vi "Drive Command Handler Temp.vi"(6 "Operator POVs":i16[](array[numeric]), 7 "Driver POVs":i16[](array[numeric]), 8 "Operator Axes":dbl[](array[numeric]), 9 "Operator Buttons":bool[](array[boolean]), 10 "Driver Buttons":bool[](array[boolean]), 11 "Driver Axes":dbl[](array[numeric])) -> ()   [LabVIEW 2019]
uses:
  Implementation/Drive Base Operations.ctl
  4946ced4-976c-43e8-b0b1-bcd015106e49.vi
  41fdccfd-133c-48c3-bd45-6bb0d7214a34.vi
  963458c1-dddb-4085-8820-b897a4c2a4ef.vi
  a950058a-1ddc-42d1-ab8e-bd80fb7a5a61.vi
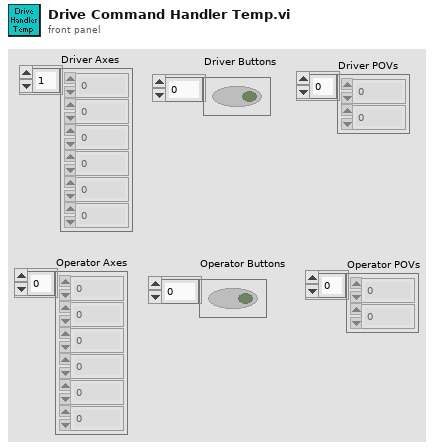
[diagram p1: front panel]
types:
  T1 = typedef "Drive Base Operations.ctl" = enum16{"Reserve", "Read Current", "Immediate", "Immediate Limelight", "Immediate Duration", "Limelight", "Manual Adjustment", "Play Path"}
  T2 = cluster{"f":T1, "Cluster":cluster{"Numeric":dbl, "Numeric 2":dbl}}
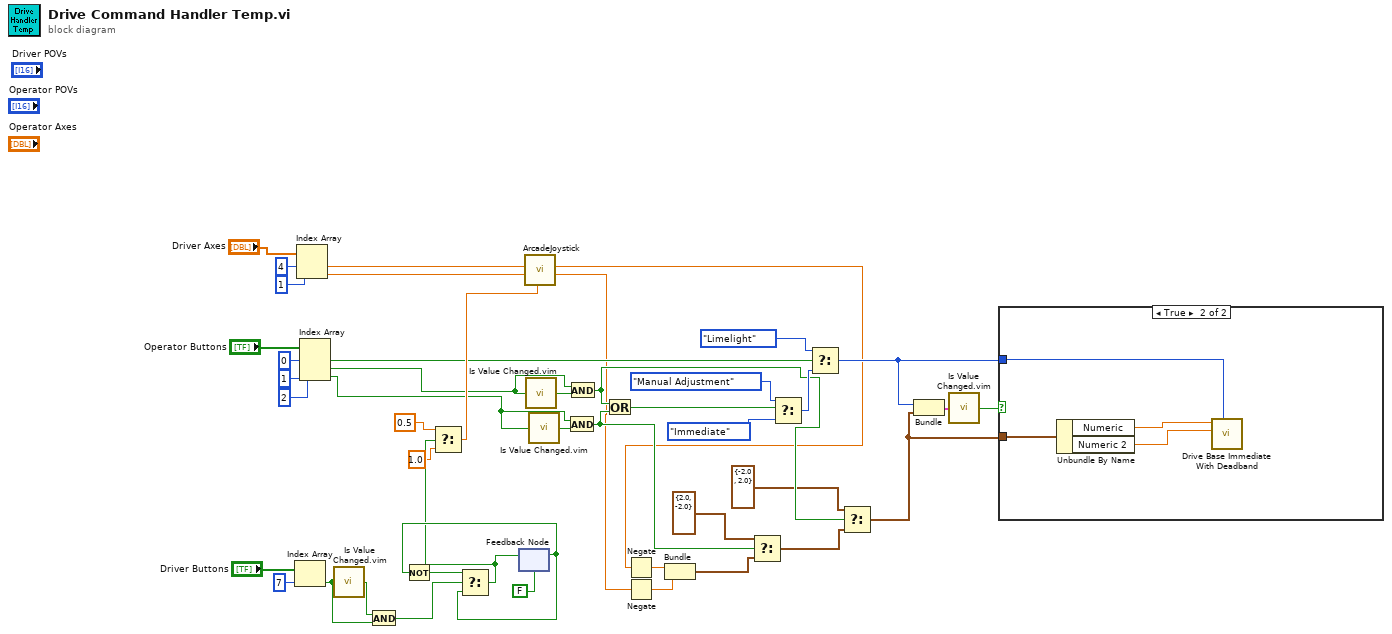
[diagram p0: block diagram]
diagram:
  n1 = Index Array(array="Driver Buttons", index=7) -> (element=w27:bool)
  n2 = Index Array(array="Driver Axes", index #1=4 ("index"), index #2=1 ("index")) -> (element #1=w36:dbl, element #2=w35:dbl)
  n3 = Index Array(array="Operator Buttons", index #1=0 ("index"), index #2=1 ("index"), index #3=2 ("index")) -> (element #1=w24:bool, element #2=w21:bool, element #3=w19:bool)
  n4 = call "Is Value Changed.vim"("value"=w27) -> ("changed or first call?"=w28:bool)
  n5 = And(x=w28, y=w27) -> (x .and. y?=w26:bool)
  n6 = feedback #1(FALSE) -> (w33:bool)
  n7 = Not(x=w33) -> (.not. x?=w32:bool)
  n8 = Select(t=w32, s=w26, f=w33) -> (s? t:f=w31:bool)
  n9 = Select(t=0.5, s=w31, f=1.0) -> (s? t:f=w25:dbl)
  n10 = feedback-in #1(w31) -> ()
  n11 = call "ArcadeJoystick.vi"("Max Output"=w25, "Y axis value"=w35, "X axis value"=w36) -> ("Right Motor Value"=w2:dbl, "Left Motor Value"=w3:dbl)  [unwired: 7 in]
  n12 = call "Is Value Changed.vim"("value"=w21) -> ("changed or first call?"=w22:bool)
  n13 = call "Is Value Changed.vim"("value"=w19) -> ("changed or first call?"=w20:bool)
  n14 = And(x=w19, y=w20) -> (x .and. y?=w8:bool)
  n15 = And(x=w21, y=w22) -> (x .and. y?=w11:bool)
  n16 = Or(x=w11, y=w8) -> (x .or. y?=w12:bool)
  n17 = Negate(x=w3) -> (-x=w1:dbl)
  n18 = Negate(x=w2) -> (-x=w4:dbl)
  n19 = Bundle(w1, w4) -> (w9:cluster{dbl, dbl})  [unwired: 1 in]
  n20 = Select(t=cluster{"Numeric":dbl, "Numeric 2":dbl} {"Numeric"=2.0, "Numeric 2"=-2.0} ("Cluster"), s=w8, f=w9) -> (s? t:f=w6:cluster{"Numeric":dbl, "Numeric 2":dbl})
  n21 = Select(t=Drive_Base_Operations."Manual Adjustment" ("Operation"), s=w12, f=Drive_Base_Operations."Immediate") -> (s? t:f=w17:T1)
  n22 = Select(t=Drive_Base_Operations."Limelight" ("Operation"), s=w24, f=w17) -> (s? t:f=w13:T1)
  n23 = Select(t=cluster{"Numeric":dbl, "Numeric 2":dbl} {"Numeric"=-2.0, "Numeric 2"=2.0} ("Cluster"), s=w11, f=w6) -> (s? t:f=w5:cluster{"Numeric":dbl, "Numeric 2":dbl})
  n24 = Bundle("f"=w13, "Cluster"=w5) -> (w15:T2)  [unwired: 1 in]
  n25 = call "Is Value Changed.vim"("value"=w15) -> ("changed or first call?"=w14:bool)
  n26 = case shown="True" w14 {
    tunnel: w13 -> [_ w49]
    tunnel: w5 -> [_ w48]
    frame False {
    }
    frame True {
      n27 = Unbundle By Name(w48) -> ("Numeric"=w47:dbl, "Numeric 2"=w46:dbl)
      n28 = call "Drive Base Immediate With Deadband.vi"("Operation"=w49, "Right Setpoint"=w46, "Left Setpoint"=w47) -> ()  [unwired: 8 in, 1 out]
    }
  }
